vi "read_Object.vi"(0 "Interface_object in":refnum<class "SwitchableDevice.lvclass">, 3 "destroy Interface (T)":bool=TRUE, 5 "error in (no error)":errorcluster) -> (14 "Interface_object out":refnum<class "SwitchableDevice.lvclass">, 16 "Object":refnum<class>, 19 "error out":errorcluster)   [LabVIEW 2018, in "SwitchableDevice.lvclass"]
doc: "<b>Auto-created method</b>\n\nReturns object that can be downcast to specific class. The downcast must be done explicitly using node <b>To More Specific Class</b> and corresponding class constant. \n\nOptionally destroys instance of the Interface (but not instance of the class)."
uses:
  SwitchableDevice.lvclass
  SwitchableDevice.lvclass/SwitchableDevice.ctl
panel:
  # "Do not edit this method"
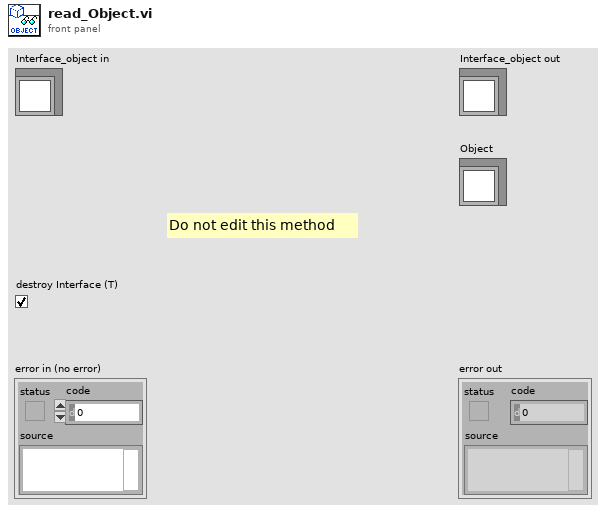
[diagram p1: front panel]
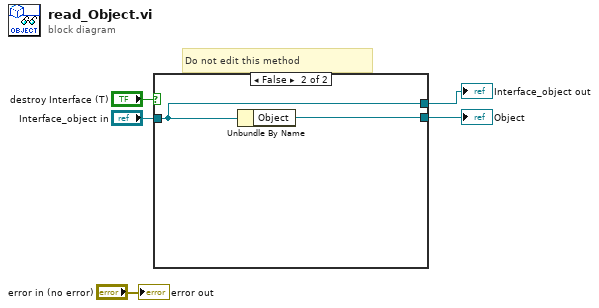
[diagram p0: block diagram]
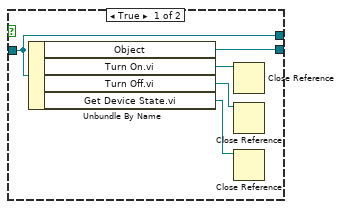
[diagram p2: hidden frame]
diagram:
  # "Do not edit this method"
  n1 = case shown="False" "destroy Interface (T)" {
    tunnel: [w10 w12] -> w3
    tunnel: "Interface_object in" -> [w10 w12]
    tunnel: [w9 w11] -> w1
    frame True {
      n2 = Unbundle By Name(w10) -> ("Object"=w9:refnum<class>, "Turn On.vi"=w8:refnum<vi>, "Turn Off.vi"=w7:refnum<vi>, "Get Device State.vi"=w6:refnum<vi>)
      n3 = Close Reference(reference=w8) -> ()  [unwired: 1 in, 1 out]
      n4 = Close Reference(reference=w7) -> ()  [unwired: 1 in, 1 out]
      n5 = Close Reference(reference=w6) -> ()  [unwired: 1 in, 1 out]
    }
    frame False {
      n6 = Unbundle By Name(w12) -> ("Object"=w11:refnum<class>)
    }
  }
  "Interface_object out" <- w3
  "Object" <- w1
  "error out" <- "error in (no error)"
